vi "test-Vision-Utils-Test2.vi"() -> (3 "All Passed":bool)   [LabVIEW 2019]
uses:
  <vilib>/Rock Robotics/WPI/ThirdParty/JAS_Junk/TrajLib/Trajectory_Library.lvlib
panel:
  out "Test 3":bool
  out "Test 2":bool
  out "Test 1":bool
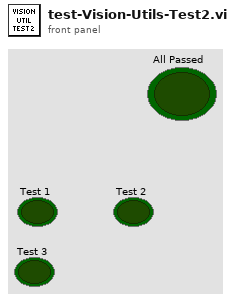
[diagram p1: front panel]
types:
  T1 = typedef "Trajectory_Library.lvlib/ROTATION2D.ctl" = cluster{"VALUE":dbl, "COS":dbl, "SIN":dbl}
  T2 = typedef "Trajectory_Library.lvlib/POSE3D.ctl" = cluster{"Translation3d":T3, "Rotation3d":T4}
  T3 = typedef "Trajectory_Library.lvlib/TRANSLATION3D.ctl" = cluster{"X":dbl, "Y":dbl, "Z":dbl}
  T4 = typedef "Trajectory_Library.lvlib/ROTATION3D.ctl" = cluster{"Q_quaternion":T5}
  T5 = typedef "Trajectory_Library.lvlib/QUATERNION.ctl" = cluster{"R":dbl, "V":dbl[]}
  T6 = typedef "Trajectory_Library.lvlib/TRANSFORM3D.ctl" = cluster{"TRANSLATION3D":T3, "ROTATION3D":T4, "XF":bool}
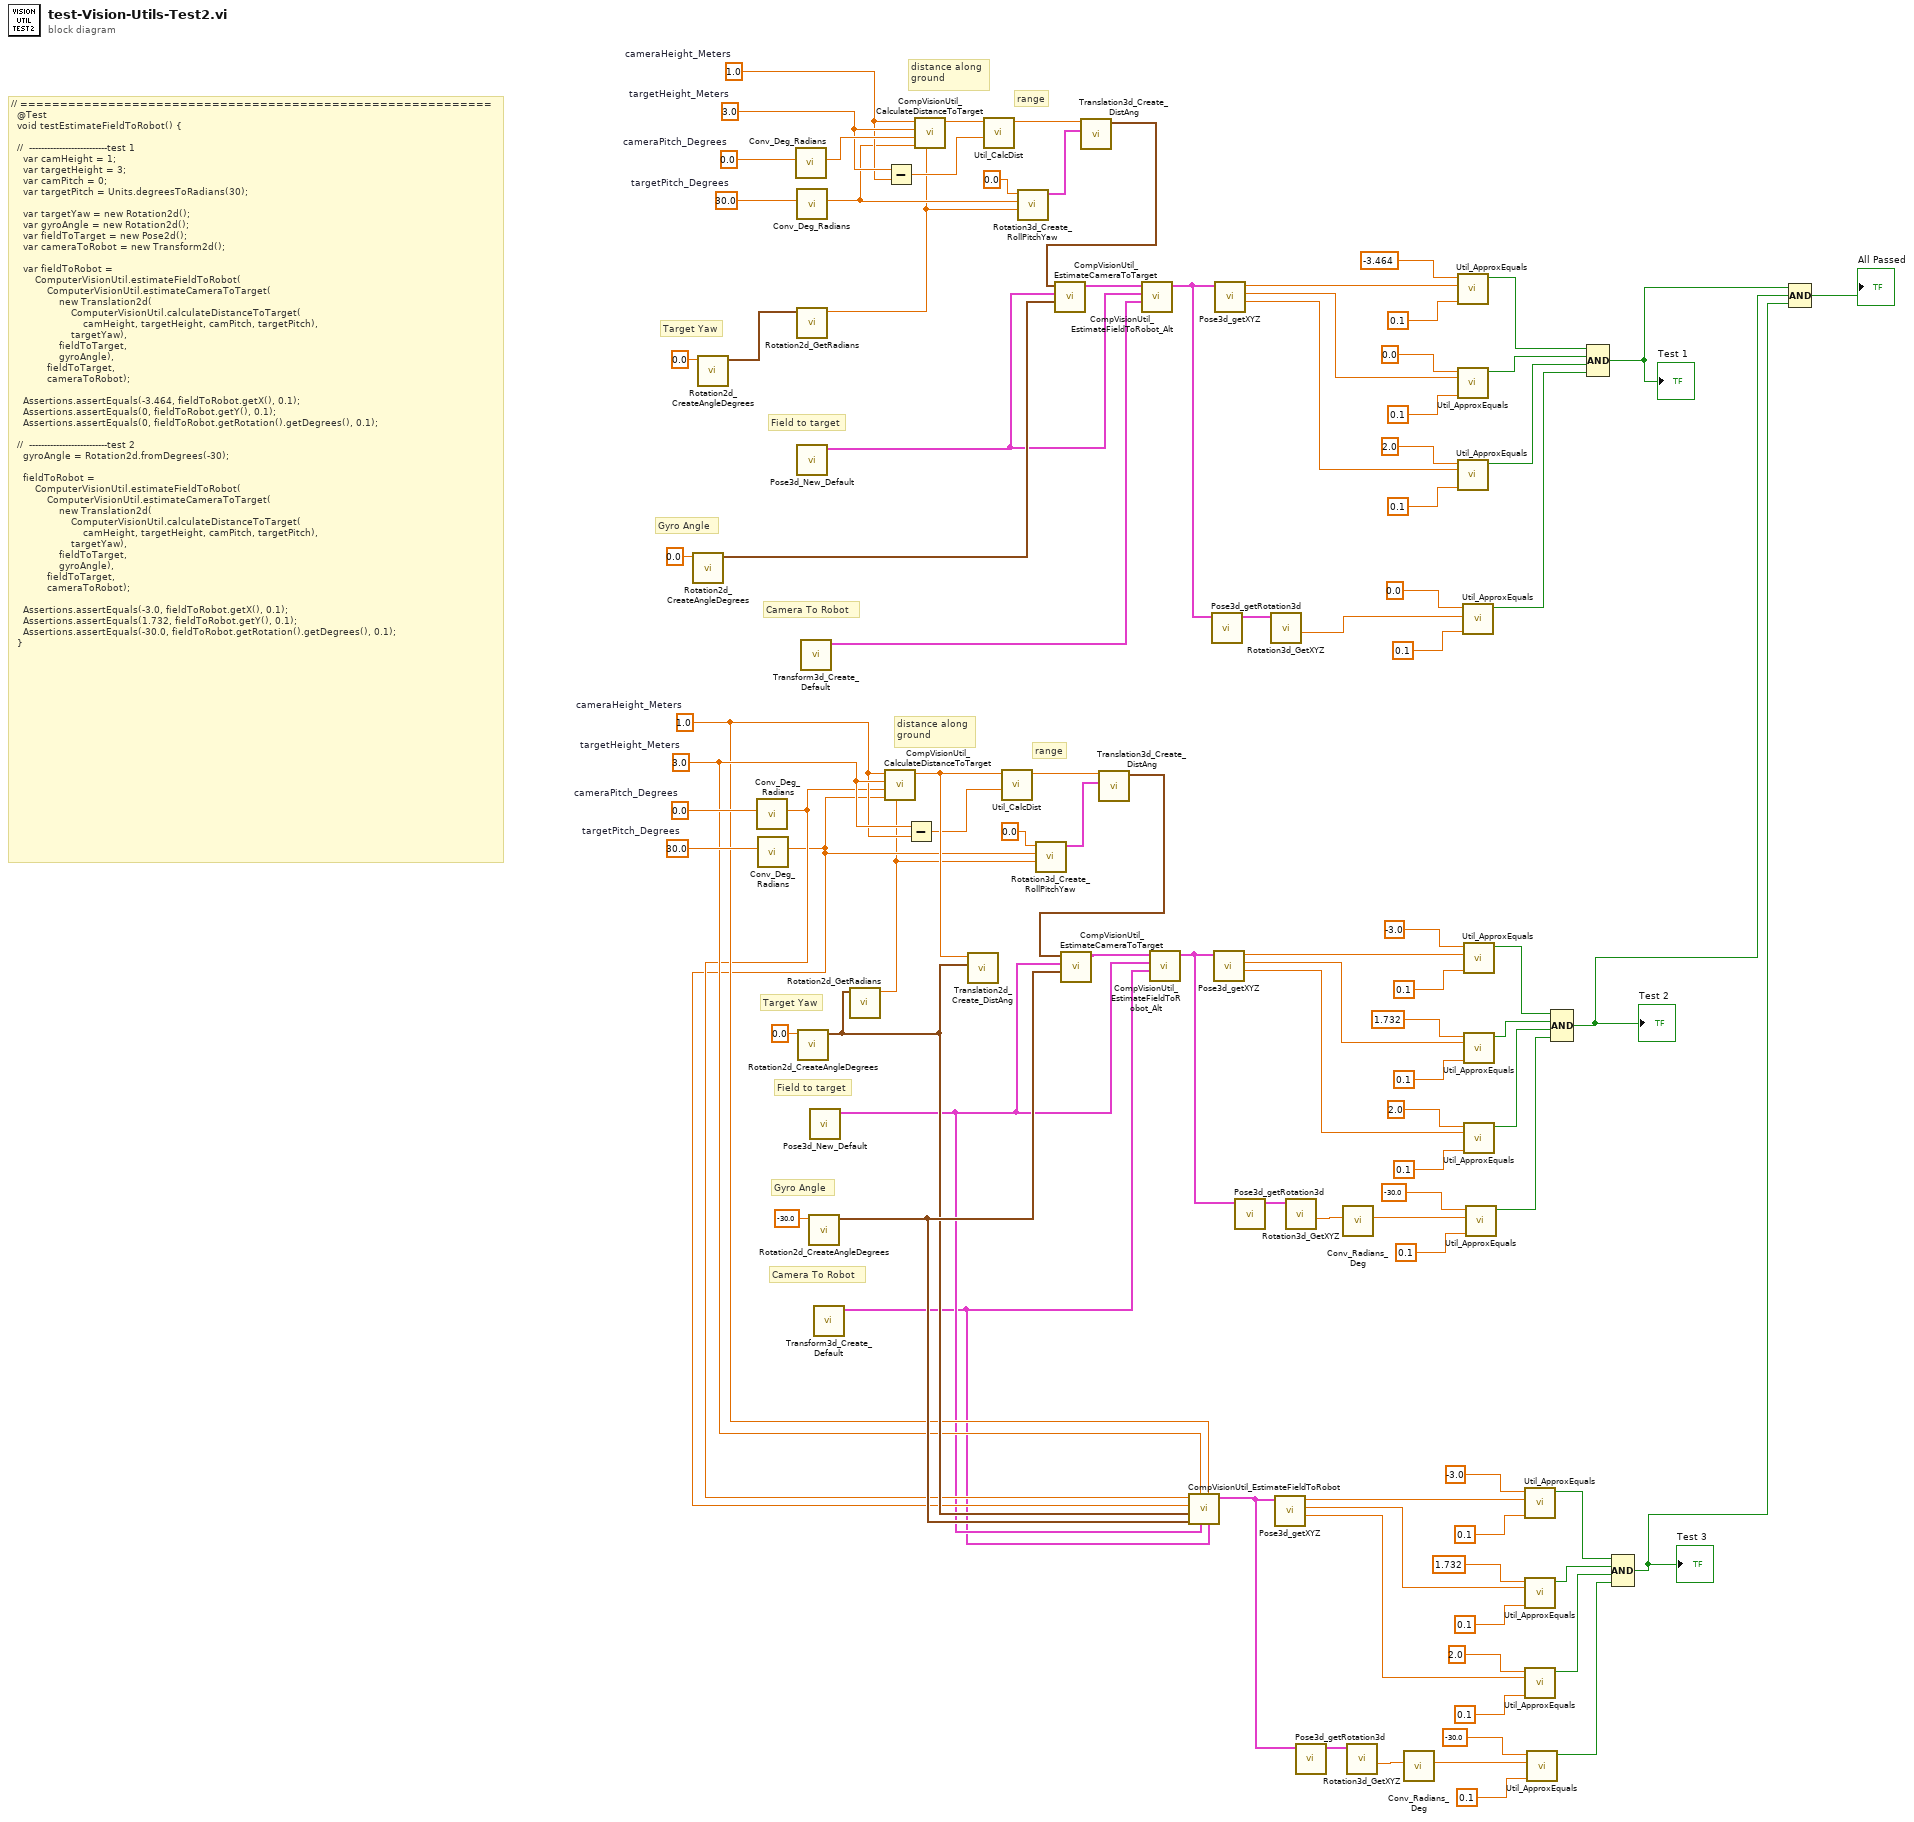
[diagram p0: block diagram]
diagram:
  w39 = 1.0  # cameraHeight_Meters
  w40 = 3.0  # targetHeight_Meters
  w70 = 0.0  # cameraPitch_Degrees
  w69 = 30.0  # targetPitch_Degrees
  w62 = 1.0  # cameraHeight_Meters
  w63 = 3.0  # targetHeight_Meters
  w97 = 0.0  # cameraPitch_Degrees
  w96 = 30.0  # targetPitch_Degrees
  # "range"
  # "distance along\nground"
  # "range"
  # "distance along\nground"
  # "Camera To Robot"
  # "Field to target"
  # "Gyro Angle"
  # "Target Yaw"
  # "Camera To Robot"
  # "Field to target"
  # "Gyro Angle"
  # "Target Yaw"
  # "// ===========================================================\n  @Test\n  void testEstimateFieldToRobot() {\n\n  //  --------------------------test 1\n    var camHeight = 1;\n    var targetHeight = 3;\n    var camPitch = 0;\n    var targetPitch = Units.degreesToRadians(30);\n\n    var targetYaw = new Rotation2d();\n    var gyroAngle = new Rotation2d();\n    var fieldToTarget = new Pose2d();\n    var cameraToRobot = new Transform2d();\n\n    var fieldToRobot =\n        ComputerVisionUtil.estimateFieldToRobot(\n            ComputerVisionUtil.estimateCameraToTarget(\n                new Translation2d(\n                    ComputerVisionUtil.calculateDistanceToTarget(\n                        camHeight, targetHeight, camPitch, targetPitch),\n                    targetYaw),\n                fieldToTarget,\n                gyroAngle),\n            fieldToTarget,\n            cameraToRobot);\n\n    Assertions.assertEquals(-3.464, fieldToRobot.getX(), 0.1);\n    Assertions.assertEquals(0, fieldToRobot.getY(), 0.1);\n    Assertions.assertEquals(0, fieldToRobot.getRotation().getDegrees(), 0.1);\n\n  //  --------------------------test 2\n    gyroAngle = Rotation2d.fromDegrees(-30);\n\n    fieldToRobot =\n        ComputerVisionUtil.estimateFieldToRobot(\n            ComputerVisionUtil.estimateCameraToTarget(\n                new Translation2d(\n                    ComputerVisionUtil.calculateDistanceToTarget(\n                        camHeight, targetHeight, camPitch, targetPitch),\n                    targetYaw),\n                fieldToTarget,\n                gyroAngle),\n            fieldToTarget,\n            cameraToRobot);\n\n    Assertions.assertEquals(-3.0, fieldToRobot.getX(), 0.1);\n    Assertions.assertEquals(1.732, fieldToRobot.getY(), 0.1);\n    Assertions.assertEquals(-30.0, fieldToRobot.getRotation().getDegrees(), 0.1);\n  }"
  n1 = call <vilib>:"Rotation2d_CreateAngleDegrees.vi"("Angle_Degrees"=0.0) -> ("ROTATION"=w92:T1)  [unwired: 10 in]
  n2 = call <vilib>:"Rotation2d_CreateAngleDegrees.vi"("Angle_Degrees"=0.0) -> ("ROTATION"=w67:T1)  [unwired: 10 in]
  n3 = call <vilib>:"Conv_Deg_Radians.vi"("Degress"=w70) -> ("Radians"=w36:dbl)  [unwired: 10 in]
  n4 = call <vilib>:"Conv_Deg_Radians.vi"("Degress"=w69) -> ("Radians"=w35:dbl)  [unwired: 10 in]
  n5 = call <vilib>:"Conv_Deg_Radians.vi"("Degress"=w97) -> ("Radians"=w95:dbl)  [unwired: 10 in]
  n6 = call <vilib>:"Conv_Deg_Radians.vi"("Degress"=w96) -> ("Radians"=w56:dbl)  [unwired: 10 in]
  n7 = call <vilib>:"Rotation2d_GetRadians.vi"("in ROTATION"=w67) -> ("AngleRadians"=w55:dbl)  [unwired: 10 in]
  n8 = call <vilib>:"Pose3d_New_Default.vi"() -> ("outPose3d"=w65:T2)  [unwired: 11 in]
  n9 = call <vilib>:"Rotation2d_CreateAngleDegrees.vi"("Angle_Degrees"=0.0) -> ("ROTATION"=w66:T1)  [unwired: 10 in]
  n10 = call <vilib>:"Transform3d_Create_Default.vi"() -> ("Transform3d"=w64:T6)  [unwired: 11 in]
  n11 = call <vilib>:"Rotation2d_CreateAngleDegrees.vi"("Angle_Degrees"=-30.0) -> ("ROTATION"=w68:T1)  [unwired: 10 in]
  n12 = call <vilib>:"Pose3d_New_Default.vi"() -> ("outPose3d"=w32:T2)  [unwired: 11 in]
  n13 = call <vilib>:"Transform3d_Create_Default.vi"() -> ("Transform3d"=w31:T6)  [unwired: 11 in]
  n14 = call <vilib>:"Rotation2d_GetRadians.vi"("in ROTATION"=w66) -> ("AngleRadians"=w34:dbl)  [unwired: 10 in]
  n15 = call <vilib>:"CompVisionUtil_CalculateDistanceToTarget.vi"("TargetYawRadians"=w34, "targetPitch_Radians"=w35, "cameraPitch_Radians"=w36, "targetHeight_Meters"=w40, "cameraHeight_Meters"=w39) -> ("DistanceToTarget_Meters"=w38:dbl)  [unwired: 6 in]
  n16 = Subtract(x=w63, y=w62) -> (x-y=w60:dbl)
  n17 = Subtract(x=w40, y=w39) -> (x-y=w37:dbl)
  n18 = call <vilib>:"CompVisionUtil_CalculateDistanceToTarget.vi"("TargetYawRadians"=w55, "targetPitch_Radians"=w56, "cameraPitch_Radians"=w95, "targetHeight_Meters"=w63, "cameraHeight_Meters"=w62) -> ("DistanceToTarget_Meters"=w61:dbl)  [unwired: 6 in]
  n19 = call <vilib>:"Translation2d_Create_DistAng.vi"("Angle"=w66, "Dist"=w38) -> ()  [unwired: 9 in, 1 out]
  n20 = call <vilib>:"Util_CalcDist.vi"("Y"=w60, "X"=w61) -> ("DIST"=w59:dbl)  [unwired: 9 in]
  n21 = call <vilib>:"Util_CalcDist.vi"("Y"=w37, "X"=w38) -> ("DIST"=w43:dbl)  [unwired: 9 in]
  n22 = call <vilib>:"Rotation3d_Create_RollPitchYaw.vi"("Yaw"=w55, "Pitch"=w56, "Roll"=0.0) -> ("Rotation3d"=w58:T4)  [unwired: 8 in]
  n23 = call <vilib>:"Rotation3d_Create_RollPitchYaw.vi"("Yaw"=w34, "Pitch"=w35, "Roll"=0.0) -> ("Rotation3d"=w42:T4)  [unwired: 8 in]
  n24 = call <vilib>:"Translation3d_Create_DistAng.vi"("Angle_Rotation3d"=w58, "Distance"=w59) -> ("TRANSLATION3D"=w54:T3)  [unwired: 9 in]
  n25 = call <vilib>:"CompVisionUtil_EstimateCameraToTarget.vi"("GyroAngle"=w92, "FieldToTarget"=w65, "CameraToTargetTranslation"=w54) -> ("EstimateCameraToTarget"=w91:T6)  [unwired: 8 in]
  n26 = call <vilib>:"Translation3d_Create_DistAng.vi"("Angle_Rotation3d"=w42, "Distance"=w43) -> ("TRANSLATION3D"=w33:T3)  [unwired: 9 in]
  n27 = call <vilib>:"CompVisionUtil_EstimateCameraToTarget.vi"("GyroAngle"=w68, "FieldToTarget"=w32, "CameraToTargetTranslation"=w33) -> ("EstimateCameraToTarget"=w79:T6)  [unwired: 8 in]
  n28 = call <vilib>:"CompVisionUtil_EstimateFieldToRobot_Alt.vi"("CameraToRobot"=w64, "FieldToTarget"=w65, "CameraToTarget"=w91) -> ("EstimatedFieldToRobot"=w53:T2)  [unwired: 8 in]
  n29 = call <vilib>:"CompVisionUtil_EstimateFieldToRobot_Alt.vi"("CameraToRobot"=w31, "FieldToTarget"=w32, "CameraToTarget"=w79) -> ("EstimatedFieldToRobot"=w29:T2)  [unwired: 8 in]
  n30 = call <vilib>:"CompVisionUtil_EstimateFieldToRobot.vi"("CameraToRobot"=w31, "cameraHeight_Meters"=w39, "FieldToTarget"=w32, "targetHeight_Meters"=w40, "GyroAngle"=w68, "TargetYaw"=w66, "targetPitch_Radians"=w35, "cameraPitch_Radians"=w36) -> ("EstimateFieldToRobot"=w2:T2)  [unwired: 3 in]
  n31 = call <vilib>:"Pose3d_getRotation3d.vi"("in Pose3d"=w53) -> ("out Rotation3d"=w46:T4)  [unwired: 10 in]
  n32 = call <vilib>:"Pose3d_getXYZ.vi"("in Pose3d"=w29) -> ("Z"=w24:dbl, "Y"=w27:dbl, "X"=w28:dbl)  [unwired: 8 in]
  n33 = call <vilib>:"Pose3d_getXYZ.vi"("in Pose3d"=w53) -> ("Z"=w48:dbl, "Y"=w51:dbl, "X"=w52:dbl)  [unwired: 8 in]
  n34 = call <vilib>:"Pose3d_getRotation3d.vi"("in Pose3d"=w29) -> ("out Rotation3d"=w30:T4)  [unwired: 10 in]
  n35 = call <vilib>:"Rotation3d_GetXYZ.vi"("in Rotation3d"=w46) -> ("Z"=w45:dbl)  [unwired: 8 in, 2 out]
  n36 = call <vilib>:"Pose3d_getXYZ.vi"("in Pose3d"=w2) -> ("Z"=w6:dbl, "Y"=w9:dbl, "X"=w10:dbl)  [unwired: 8 in]
  n37 = call <vilib>:"Rotation3d_GetXYZ.vi"("in Rotation3d"=w30) -> ("Z"=w21:dbl)  [unwired: 8 in, 2 out]
  n38 = call <vilib>:"Pose3d_getRotation3d.vi"("in Pose3d"=w2) -> ("out Rotation3d"=w11:T4)  [unwired: 10 in]
  n39 = call <vilib>:"Conv_Radians_Deg.vi"("Radians"=w21) -> ("Degrees"=w72:dbl)  [unwired: 10 in]
  n40 = call <vilib>:"Rotation3d_GetXYZ.vi"("in Rotation3d"=w11) -> ("Z"=w3:dbl)  [unwired: 8 in, 2 out]
  n41 = call <vilib>:"Conv_Radians_Deg.vi"("Radians"=w3) -> ("Degrees"=w12:dbl)  [unwired: 10 in]
  n42 = call <vilib>:"Util_ApproxEquals.vi"("Tolerance"=0.1, "Value 2"=w52, "Value 1"=-3.464 ("y")) -> ("ApproxEquals"=w86:bool)  [unwired: 8 in]
  n43 = call <vilib>:"Util_ApproxEquals.vi"("Tolerance"=0.1, "Value 2"=w51, "Value 1"=0.0 ("y")) -> ("ApproxEquals"=w85:bool)  [unwired: 8 in]
  n44 = call <vilib>:"Util_ApproxEquals.vi"("Tolerance"=0.1, "Value 2"=w48, "Value 1"=2.0 ("y")) -> ("ApproxEquals"=w47:bool)  [unwired: 8 in]
  n45 = call <vilib>:"Util_ApproxEquals.vi"("Tolerance"=0.1, "Value 2"=w45, "Value 1"=0.0 ("y")) -> ("ApproxEquals"=w44:bool)  [unwired: 8 in]
  n46 = call <vilib>:"Util_ApproxEquals.vi"("Tolerance"=0.1, "Value 2"=w28, "Value 1"=-3.0 ("y")) -> ("ApproxEquals"=w74:bool)  [unwired: 8 in]
  n47 = call <vilib>:"Util_ApproxEquals.vi"("Tolerance"=0.1, "Value 2"=w27, "Value 1"=1.732 ("y")) -> ("ApproxEquals"=w73:bool)  [unwired: 8 in]
  n48 = call <vilib>:"Util_ApproxEquals.vi"("Tolerance"=0.1, "Value 2"=w24, "Value 1"=2.0 ("y")) -> ("ApproxEquals"=w22:bool)  [unwired: 8 in]
  n49 = call <vilib>:"Util_ApproxEquals.vi"("Tolerance"=0.1, "Value 2"=w72, "Value 1"=-30.0 ("y")) -> ("ApproxEquals"=w23:bool)  [unwired: 8 in]
  n50 = call <vilib>:"Util_ApproxEquals.vi"("Tolerance"=0.1, "Value 2"=w10, "Value 1"=-3.0 ("y")) -> ("ApproxEquals"=w14:bool)  [unwired: 8 in]
  n51 = call <vilib>:"Util_ApproxEquals.vi"("Tolerance"=0.1, "Value 2"=w9, "Value 1"=1.732 ("y")) -> ("ApproxEquals"=w13:bool)  [unwired: 8 in]
  n52 = call <vilib>:"Util_ApproxEquals.vi"("Tolerance"=0.1, "Value 2"=w6, "Value 1"=2.0 ("y")) -> ("ApproxEquals"=w4:bool)  [unwired: 8 in]
  n53 = call <vilib>:"Util_ApproxEquals.vi"("Tolerance"=0.1, "Value 2"=w12, "Value 1"=-30.0 ("y")) -> ("ApproxEquals"=w5:bool)  [unwired: 8 in]
  n54 = Compound Arithmetic op=AND(w74, w73, w22, w23) -> (w71:bool)
  "Test 2" <- w71
  n55 = Compound Arithmetic op=AND(w86, w85, w47, w44) -> (w84:bool)
  "Test 1" <- w84
  n56 = Compound Arithmetic op=AND(w14, w13, w4, w5) -> (w1:bool)
  "Test 3" <- w1
  n57 = Compound Arithmetic op=AND(w84, w71, w1) -> (→"All Passed":bool)
